vi "Init Loggers.vi"(8 "error in (no error)":errorcluster, 11 "Logger Mananger in":refnum<class "Logger Mananger.lvclass">) -> (0 "error out":errorcluster, 3 "Logger Mananger out":refnum<class "Logger Mananger.lvclass">)   [LabVIEW 2020, in "Logging.lvlib" / "Logger Mananger.lvclass"]
uses:
  Logger Mananger.lvclass
  Logger Mananger.lvclass/Logger Mananger.ctl
  Logging.lvlib
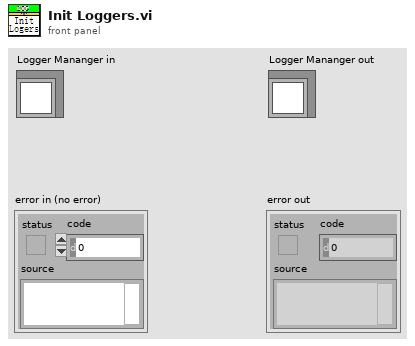
[diagram p1: front panel]
types:
  T1 = typedef "Logging.lvlib/Log Setting.ctl" = cluster{"Msg Pattern":string, "Time Format":string, "Logges":T2[]}
  T2 = typedef "Logging.lvlib/Logger Setting.ctl" = cluster{"Log Option":T3, "Log Level":T4}
  T3 = typedef "Logging.lvlib/Log Option.ctl" = string
  T4 = typedef "Logging.lvlib/Log Level.ctl" = enum16{"Debug", "Info", "Warn", "Error"}
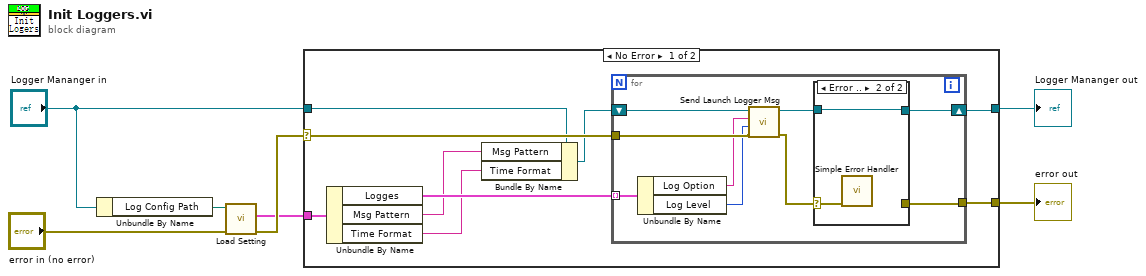
[diagram p0: block diagram]
diagram:
  n1 = Unbundle By Name("Logger Mananger in") -> ("Log Config Path"=w1:path)
  n2 = call "Load Setting.vi"("error in (no error)"="error in (no error)", "Log Config Path"=w1) -> ("error out"=w4:errorcluster, "Setting"=w3:T1)  [unwired: 8 in]
  n3 = case shown="No Error" w4 {
    selector: w4 -> [w14 w31]
    tunnel: [w12 w31] -> w7
    tunnel: [w13 w30] -> w6
    tunnel: "Logger Mananger in" -> [w11 w30]
    tunnel: w3 -> [w16 _]
    frame No Error {
      n4 = Unbundle By Name(w16) -> ("Logges"=w15:T2[], "Msg Pattern"=w9:string, "Time Format"=w8:string)
      n5 = Bundle By Name(cluster=w11, "Msg Pattern"=w9, "Time Format"=w8) -> (w10:refnum<class "Logger Mananger.lvclass">)
      n6 = for {
        tunnel: w15 -> [w25] mode=indexing
        tunnel: w14 -> [w20]
        shift-right: [w24] -> w13
        shift-left: w10 -> [w22]
        tunnel: [w23] -> w12
        n7 = Unbundle By Name(w25) -> ("Log Option"=w18:T3, "Log Level"=w17:T4)
        n8 = call "Send Launch Logger Msg.vi"("error in (no error)"=w20, "Log Level"=w17, "Logger Name"=w18, "Logger Mananger in"=w22) -> ("error out"=w19:errorcluster, "Logger Mananger out"=w21:refnum<class "Logger Mananger.lvclass">)  [unwired: 6 in]
        n9 = case shown="Error .." w19 {
          selector: w19 -> [w27 w28]
          tunnel: w21 -> [w26 w29]
          tunnel: [w26 w29] -> w24
          tunnel: [w27 _] -> w23
          frame No Error {
          }
          frame Error {
            n10 = call <vilib>:"Simple Error Handler.vi"("error in (no error)"=w28) -> ()  [unwired: 4 in, 5 out]
          }
        }
      }
    }
    frame Error {
    }
  }
  "error out" <- w7
  "Logger Mananger out" <- w6
